vi "trigger-loop.vi"(8 "错误输入（无错误）":errorcluster, 11 "Status":T1 {"Setting"."X Pos." scale=-2.0..2.0; "Setting"."Y Pos." scale=-2.0..2.0}) -> (0 "error out":errorcluster={"status"=TRUE, "code"=-200099, "source"="DAQmx Create Channel (CO-Pulse Generation-Time).vi:7440001<append>\n<B>任务名称: </B>_unnamedTask<60A>"} caption="错误输出")   [LabVIEW 2013]
uses:
  init & communication/init-status.ctl
  init & communication/Setting.ctl
  init & communication/event-package.ctl
  init & communication/Event1.ctl
  init & communication/data-package.ctl
  init & communication/Event.ctl
  <vilib>/DAQmx/create/channels.llb/DAQmx Create Channel (CO-Pulse Generation-Time).vi
  <vilib>/DAQmx/configure/timing.llb/DAQmx Timing (Implicit).vi
  <resource>/objmgr/daqmx.rc
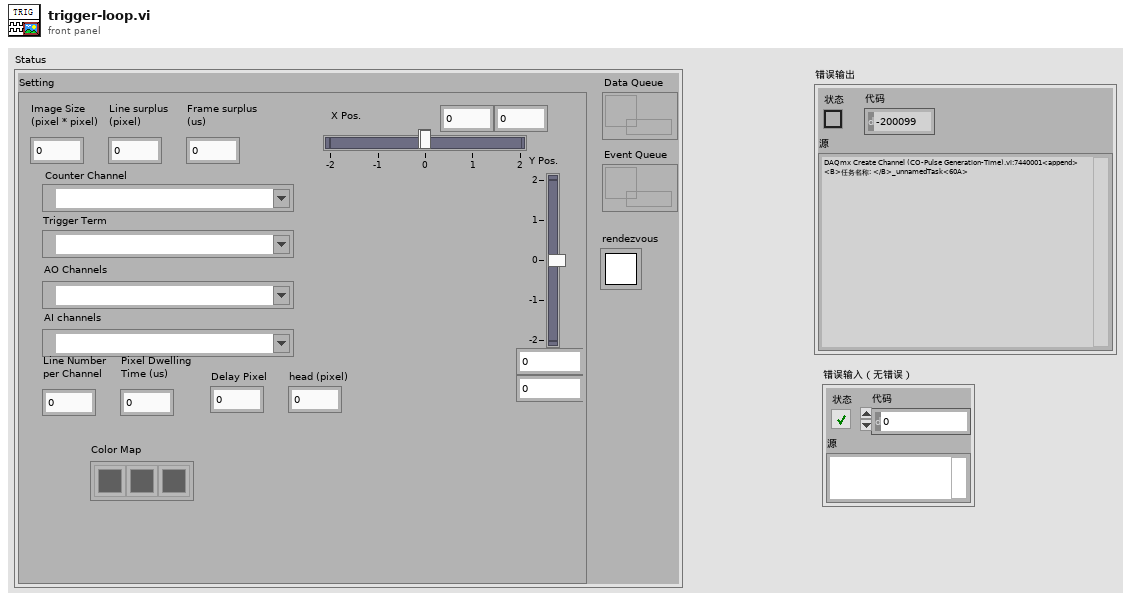
[diagram p1: front panel]
types:
  T1 = typedef "init-status.ctl" = cluster{"Setting":T2, "Event Queue":refnum<queue>, "Data Queue":refnum<queue>, "rendezvous":T3}
  T2 = typedef "Setting.ctl" = cluster{"Image Size\n(pixel * pixel)":i32, "Counter Channel":tag, "Trigger Term":tag, "AO Channels":tag, "Y Pos.":cluster{dbl, dbl}, "X Pos.":cluster{dbl, dbl}, "Line surplus\n(pixel)":i32, "Frame surplus\n(us)":i32, "AI channels":tag, "Line Number\nper Channel":i32, "Delay Pixel":i32, "Pixel Dwelling\nTime (us)":i32, "Color Map":u32[], "head (pixel)":i32}
  T3 = typedef "Rendezvous RefNum" = refnum<k1>
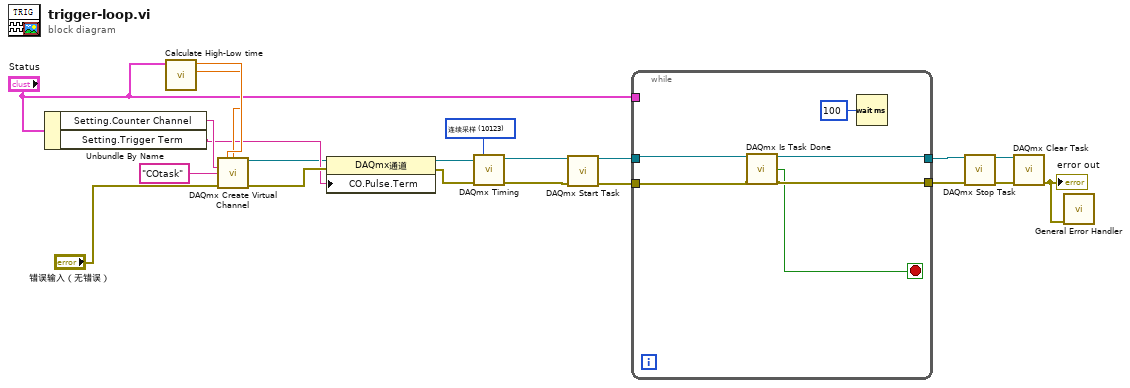
[diagram p0: block diagram]
diagram:
  w21 = 10123 items=["有限采样"=10178, "连续采样"=10123, "硬件定时单点"=12522] ("sample mode")
  n1 = Unbundle By Name("Status") -> ("Setting.Counter Channel"=w9:tag, "Setting.Trigger Term"=w6:tag)
  n2 = call "Calculate High-Low time.vi"("Status"="Status") -> ("low time"=w7:dbl, "high time"=w8:dbl)  [unwired: 9 in]
  n3 = call-poly <vilib>:"DAQmx Create Virtual Channel.vi"("high time"=w8, "low time"=w7, "counter"=w9, "name to assign"="COtask", "error in"="错误输入（无错误）") -> ("task out"=w2:refnum<k21>, "error out"=w20:errorcluster)  [unwired: 9 in]
  n4 = property class="DAQmx通道"(reference=w2, error in=w20, "CO.Pulse.Term"=w6) -> (reference out=w19:refnum<k21>, error out=w18:errorcluster)
  n5 = call-poly <vilib>:"DAQmx Timing.vi"("task/channels in"=w19, "sample mode"=w21, "error in"=w18) -> ("task out"=w17:refnum<k21>, "error out"=w1:errorcluster)  [unwired: 11 in]
  n6 = call <vilib>:"DAQmx Start Task.vi"("task/channels in"=w17, "error in"=w1) -> ("task out"=w16:refnum<k21>, "error out"=w15:errorcluster)  [unwired: 12 in]
  n7 = while {
    tunnel: w16 -> [w25]
    tunnel: w15 -> [w27]
    tunnel: "Status" -> [_]
    tunnel: [w24] -> w12
    tunnel: [w26] -> w11
    stop <- w23 stop-if-true
    n8 = call <vilib>:"DAQmx Is Task Done.vi"("task/channels in"=w25, "error in"=w27) -> ("task out"=w24:refnum<k21>, "task done?"=w23:bool, "error out"=w26:errorcluster)  [unwired: 11 in]
    n9 = Wait (ms)(milliseconds to wait=u32 100 ("等待时间（毫秒）")) -> ()  [unwired: 1 out]
  }
  n10 = call <vilib>:"DAQmx Stop Task.vi"("task/channels in"=w12, "error in"=w11) -> ("task out"=w14:refnum<k21>, "error out"=w13:errorcluster)  [unwired: 12 in]
  n11 = call <vilib>:"DAQmx Clear Task.vi"("task in"=w14, "error in"=w13) -> ("error out"=w4:errorcluster)  [unwired: 13 in]
  "error out" <- w4
  n12 = call <vilib>:"General Error Handler.vi"("error in (no error)"=w4) -> ()  [unwired: 10 in, 5 out]
